vi "Create All Events.vi"(8 "error in (no error)":errorcluster) -> (0 "error out":errorcluster, 3 "Events":T1)   [LabVIEW 2023, in "HAF.lvlib"]
doc: "Create an instance of each event understood by the framework. Stop, Pause, Resume, Done."
uses:
  HAF.lvlib
  All Events.ctl
  Stop Event.ctl
  Event Data.ctl
  Pause Event.ctl
  Resume Event.ctl
  Done Event.ctl
  Injection Event.ctl
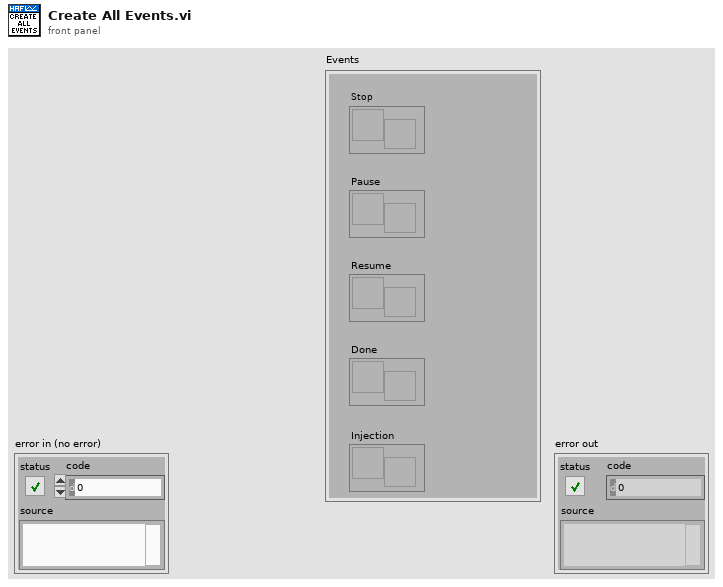
[diagram p1: front panel]
types:
  T1 = typedef "HAF.lvlib/All Events.ctl" = cluster{"Stop":T2, "Pause":T3, "Resume":T4, "Done":T5, "Injection":T6}
  T2 = typedef "HAF.lvlib/Stop Event.ctl" = refnum<user-event>
  T3 = typedef "HAF.lvlib/Pause Event.ctl" = refnum<user-event>
  T4 = typedef "HAF.lvlib/Resume Event.ctl" = refnum<user-event>
  T5 = typedef "HAF.lvlib/Done Event.ctl" = refnum<user-event>
  T6 = typedef "HAF.lvlib/Injection Event.ctl" = refnum<user-event>
  T7 = typedef "HAF.lvlib/Event Data.ctl" = cluster{"Raiser Name":string, "Raiser Id":string, "Event Data":variant}
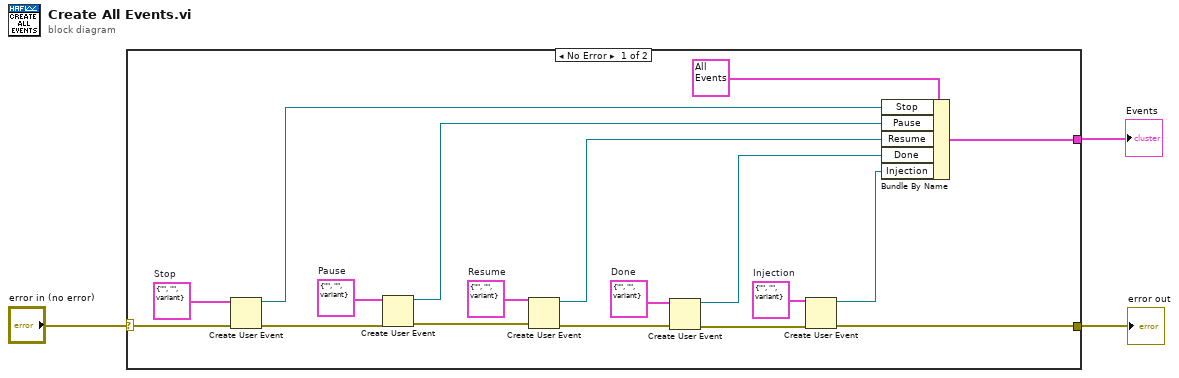
[diagram p0: block diagram]
diagram:
  n1 = case shown="No Error" "error in (no error)" {
    selector: "error in (no error)" -> [w20 w22]
    tunnel: [w8 _] -> w1
    tunnel: [w6 w22] -> w2
    frame No Error {
      w5 = T7 {"Raiser Name"="", "Raiser Id"="", "Event Data"=variant}  # Injection
      w14 = T7 {"Raiser Name"="", "Raiser Id"="", "Event Data"=variant}  # Done
      w17 = T7 {"Raiser Name"="", "Raiser Id"="", "Event Data"=variant}  # Resume
      w19 = T7 {"Raiser Name"="", "Raiser Id"="", "Event Data"=variant}  # Pause
      w21 = T7 {"Raiser Name"="", "Raiser Id"="", "Event Data"=variant}  # Stop
      n2 = Create User Event(user event datatype=w21, error in=w20) -> (user event=w12:refnum<user-event>, error out=w18:errorcluster)
      n3 = Create User Event(user event datatype=w19, error in=w18) -> (user event=w11:refnum<user-event>, error out=w16:errorcluster)
      n4 = Create User Event(user event datatype=w17, error in=w16) -> (user event=w10:refnum<user-event>, error out=w15:errorcluster)
      n5 = Create User Event(user event datatype=w14, error in=w15) -> (user event=w9:refnum<user-event>, error out=w7:errorcluster)
      n6 = Create User Event(user event datatype=w5, error in=w7) -> (user event=w4:refnum<user-event>, error out=w6:errorcluster)
      n7 = Bundle By Name(cluster=T1 {"Stop"=refnum, "Pause"=refnum, "Resume"=refnum, "Done"=refnum, "Injection"=refnum} ("Events"), "Stop"=w12, "Pause"=w11, "Resume"=w10, "Done"=w9, "Injection"=w4) -> (w8:T1)
    }
    frame Error {
    }
  }
  "error out" <- w2
  "Events" <- w1
